vi "Convert Temperature.vi"(9 "AutoZero":dbl, 10 "CJC":dbl, 11 "TC Input":dbl[](array[numeric])) -> (3 "Temperature":dbl[](array[numeric]))   [LabVIEW 2017, in "Controller.lvlib" / "gController.lvclass"]
uses:
  gController.lvclass
  C:/Program Files (x86)/National Instruments/LabVIEW 2017/examples/CompactRIO/Shared/cRIO Convert Thermocouple Readings.llb/Thermocouple Type.ctl
  C:/Program Files (x86)/National Instruments/LabVIEW 2017/examples/CompactRIO/Module Specific/NI 9213/NI 9213 Support Files.llb/NI 9213 Convert to Temperature (Calibrated).vi
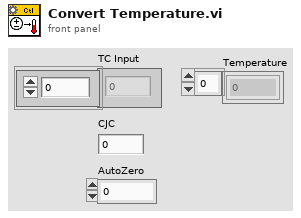
[diagram p1: front panel]
types:
  T1 = typedef "Thermocouple Type.ctl" = u16
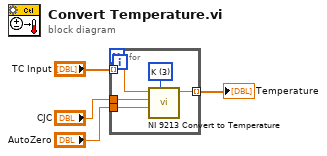
[diagram p0: block diagram]
diagram:
  n1 = for {
    tunnel: "TC Input" -> [w7] mode=indexing
    tunnel: "AutoZero" -> [w9]
    tunnel: "CJC" -> [w8]
    tunnel: [w6] -> w1 mode=indexing
    w5 = T1 3 items=["B", "E", "J", "K", "R", "S", "T", "N"] ("ThermocoupleType")
    n2 = call-poly "NI 9213 Convert to Temperature.vi"("ThermocoupleType"=w5, "AutoZero"=w9, "CJC"=w8, "TC Input"=w7) -> ("Thermocouple Temperature"=w6:dbl)  [unwired: 1 in, 6 out]
  }
  "Temperature" <- w1
